vi "format set align.vi"(8 "error in (no error)":errorcluster, 10 "alignment":u8, 11 "format":u32) -> (0 "error out":errorcluster)   [LabVIEW 8.6]
doc: "void format_set_align(lxw_format format, uint8_t alignment);"
uses:
  pending_lvxlsxwriter/xlsxwriter.dll
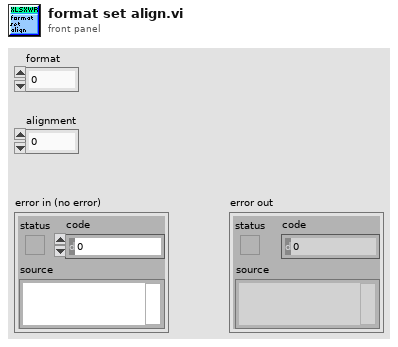
[diagram p1: front panel]
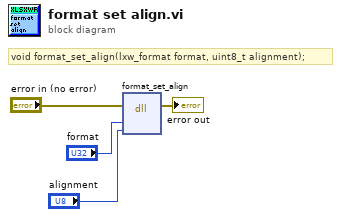
[diagram p0: block diagram]
diagram:
  # "void format_set_align(lxw_format format, uint8_t alignment);"
  n1 = dll-call lib="C:/Users/WDAGUtilityAccount/Desktop/pending_lvxlsxwriter/xlsxwriter.*" fn="format_set_align"(error in="error in (no error)", "format"="format", "alignment"="alignment") -> (error out=→"error out":errorcluster)  [unwired: 5 in, 1 out]
